vi "Epoch.DecomposeFractional.vi"(11 "Fractional in":dbl) -> (1 "Fractional":dbl, 3 "Integer":i32)   [LabVIEW 2013]
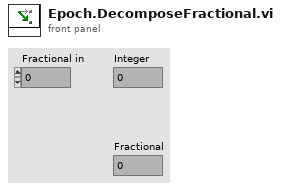
[diagram p1: front panel]
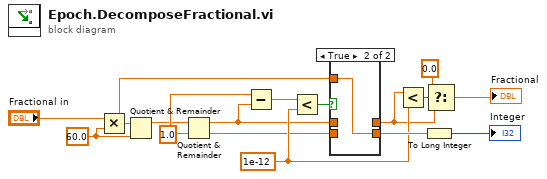
[diagram p0: block diagram]
diagram:
  w13 = 1e-12 ("y")
  w8 = 1.0 ("y")
  w2 = 60.0 ("x")
  n1 = Multiply(x="Fractional in", y=w2) -> (x*y=w5:dbl)
  n2 = Quotient & Remainder(x=w5, y=w2) -> (x-y*floor(x/y)=w4:dbl)  [unwired: 1 out]
  n3 = Quotient & Remainder(x=w4, y=w8) -> (x-y*floor(x/y)=w9:dbl, floor(x/y)=w6:dbl)
  n4 = Subtract(x=w8, y=w9) -> (x-y=w7:dbl)
  n5 = Less?(x=w7, y=w13) -> (x < y?=w3:bool)
  n6 = case shown="True" w3 {
    tunnel: [w18 w19] -> w15
    tunnel: w6 -> [w18 _]
    tunnel: w9 -> [w17 _]
    tunnel: [w17 _] -> w12
    tunnel: w5 -> [_ w19]
    frame False {
    }
    frame True {
    }
  }
  n7 = Less?(x=w12, y=w13) -> (x < y?=w10:bool)
  n8 = To Long Integer(number=w15) -> (32bit integer=→"Integer":i32)
  n9 = Select(t=0.0 ("y"), s=w10, f=w12) -> (s? t:f=→"Fractional":dbl)
